vi "PostCopyScripting.vi"(10 "MetaDataObj":refnum<class "MetaDataObj.lvclass">, 11 "User Project":refnum<vi>) -> ()   [LabVIEW 2020, in "SBMetaDataObj.lvclass"]
uses:
  SBMetaDataObj.lvclass
  SBMetaDataObj.lvclass/SBMetaDataObj.ctl
  <resource>/dialog/NewProjectWizard/MetaDataObj/MetaDataObj.lvclass
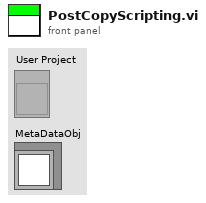
[diagram p1: front panel]
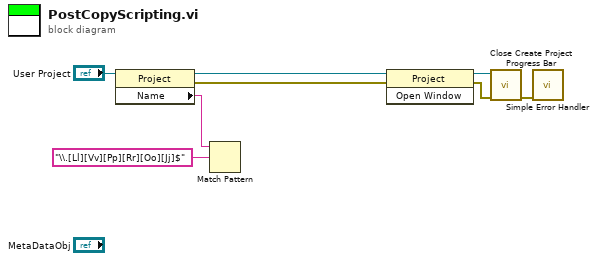
[diagram p0: block diagram]
diagram:
  n1 = property class="Project"(reference="User Project") -> (reference out=w2:refnum<vi>, error out=w1:errorcluster, "Name"=w8:string)  [unwired: 1 in]
  n2 = Match Pattern(string=w8, regular expression="\\.[Ll][Vv][Pp][Rr][Oo][Jj]$") -> ()  [unwired: 1 in, 4 out]
  n3 = invoke class="Project" method="Open Window"(reference=w2, error in=w1) -> (reference out=w5:refnum<vi>, error out=w4:errorcluster)  [unwired: 1 in, 1 out]
  n4 = call <resource>:"Close Create Project Progress Bar.vi"("error in (no error)"=w4, "Project"=w5) -> ("error out"=w3:errorcluster)  [unwired: 8 in, 1 out]
  n5 = call <vilib>:"Simple Error Handler.vi"("error in (no error)"=w3) -> ()  [unwired: 4 in, 5 out]
